vi "DG4DG1ZGeneral.vi"() -> ()   [LabVIEW 2020]
panel:
  out "output control error":errorcluster
  out "configure error out":errorcluster
  in  "Output 2":bool
  in  "Output 1":bool
  in  "Waveform Function":u16(ring)=1 items=["Sine", "Square", "Ramp", "Pulse", "Noise", "DC", "User"]
  in  "Channel Selection":u16(ring) items=["Channel 1", "Channel 2"]
  in  "Frequency (1000 Hz)":dbl=1000.0
  in  "Unit (0: Vpp)":u16(ring) items=["Vpp", "Vrms", "dB"]
  in  "DC Offset (0.00 V)":dbl
  in  "Amplitude (1)":dbl=1.0
  in  "?":bool
  in  "?":bool
  in  "VISA resource name":refnum<visa-resource-name>
  # "Rigol Technologies DG4/DG1Z General"
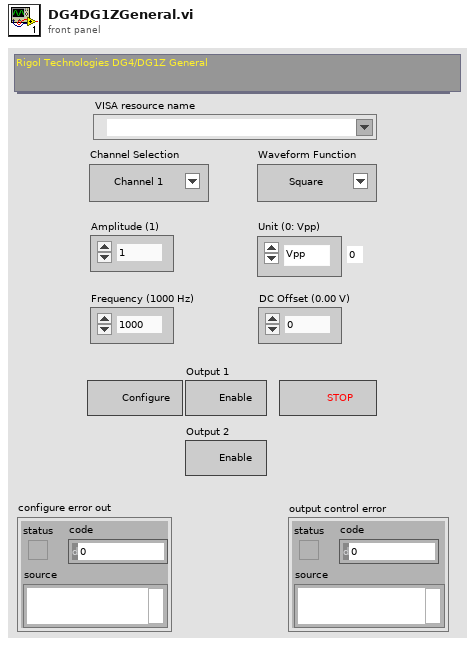
[diagram p1: front panel]
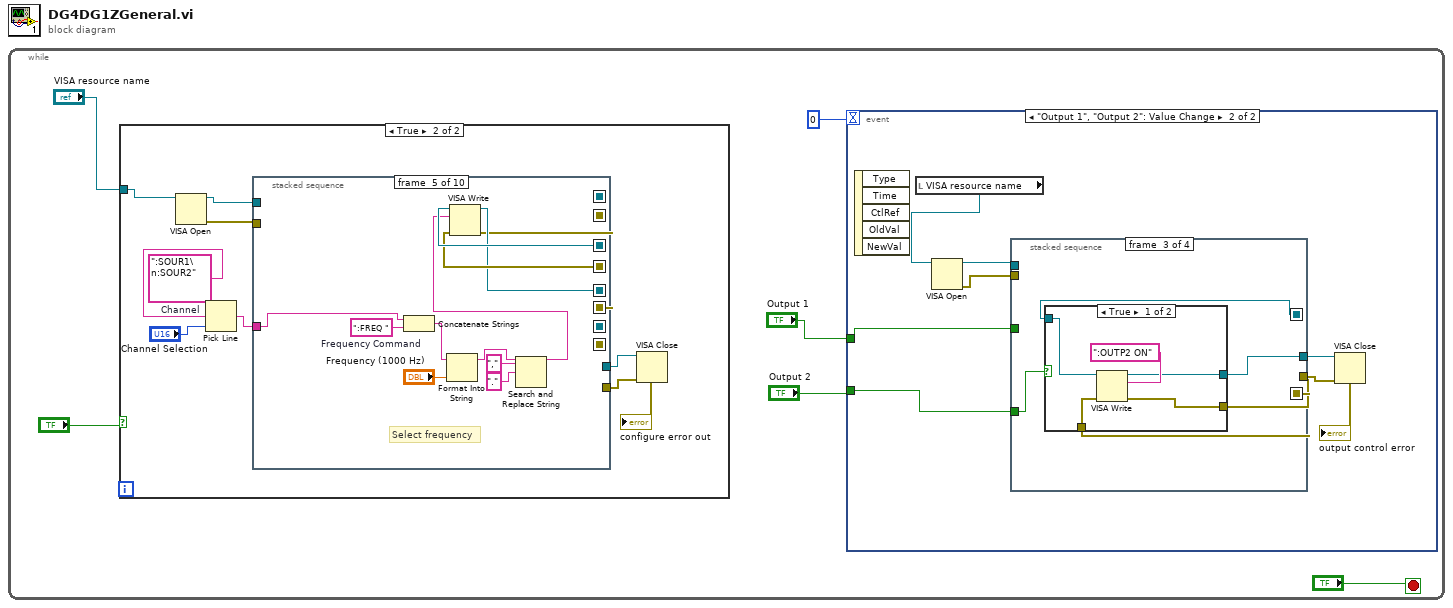
[diagram p0: block diagram]
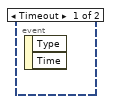
[diagram p2: hidden frame]
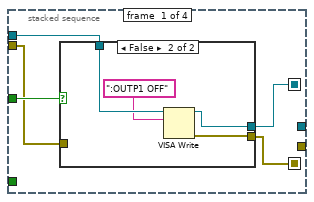
[diagram p3: hidden frame]
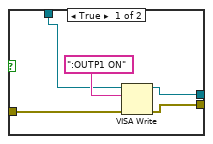
[diagram p4: hidden frame]
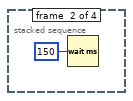
[diagram p5: hidden frame]
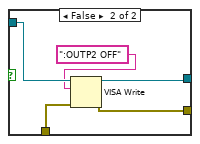
[diagram p6: hidden frame]
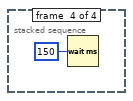
[diagram p7: hidden frame]
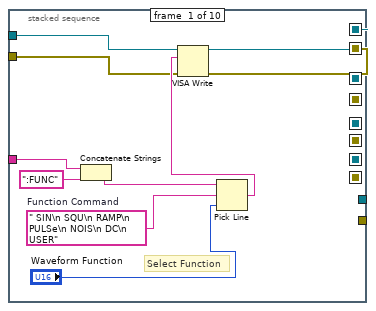
[diagram p9: hidden frame]
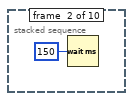
[diagram p10: hidden frame]
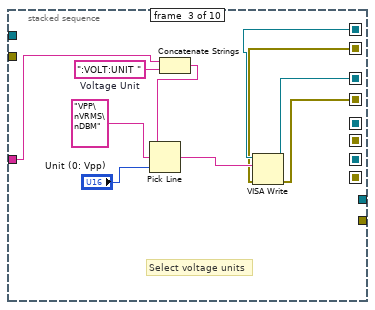
[diagram p11: hidden frame]
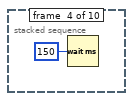
[diagram p12: hidden frame]
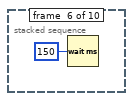
[diagram p13: hidden frame]
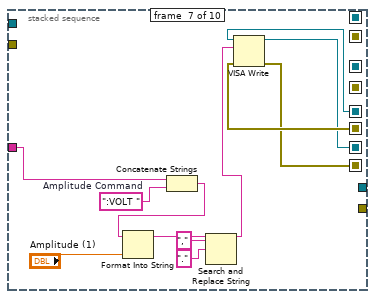
[diagram p14: hidden frame]
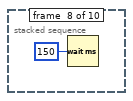
[diagram p15: hidden frame]
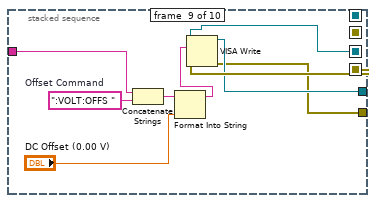
[diagram p16: hidden frame]
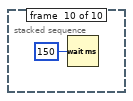
[diagram p17: hidden frame]
diagram:
  n1 = while {
    stop <- "?" stop-if-true
    n2 = case shown="True" "?" {
      tunnel: "VISA resource name" -> [_ w53]
      frame False {
      }
      frame True {
        w46 = ":SOUR1\n:SOUR2"  # Channel
        n3 = VISA Open(VISA resource name=w53) -> (VISA resource name=w52:refnum<visa-resource-name>, error out=w54:errorcluster)  [unwired: 4 in]
        n4 = Pick Line(multi-line string=w46, line index="Channel Selection") -> (output string=w48:string)  [unwired: 1 in]
        n5 = stacked-sequence {
          seq-local: [w58 _ _ _ _ _ _ _ _ _] -> [_ _ w70 _ _ _ _ _ _ _]
          seq-local: [w59 _ _ _ _ _ _ _ _ _] -> [_ _ w69 _ _ _ _ _ _ _]
          seq-local: [_ _ w68 _ _ _ _ _ _ _] -> [_ _ _ _ w85 _ _ _ _ _]
          seq-local: [_ _ w67 _ _ _ _ _ _ _] -> [_ _ _ _ w84 _ _ _ _ _]
          seq-local: [_ _ _ _ w83 _ _ _ _ _] -> [_ _ _ _ _ _ w98 _ _ _]
          seq-local: [_ _ _ _ w82 _ _ _ _ _] -> [_ _ _ _ _ _ w97 _ _ _]
          seq-local: [_ _ _ _ _ _ w96 _ _ _] -> [_ _ _ _ _ _ _ _ w107 _]
          seq-local: [_ _ _ _ _ _ w95 _ _ _] -> [_ _ _ _ _ _ _ _ w106 _]
          tunnel: w52 -> [w63 _ _ _ _ _ _ _ _ _]
          tunnel: w54 -> [w62 _ _ _ _ _ _ _ _ _]
          tunnel: [_ _ _ _ _ _ _ _ w105 _] -> w51
          tunnel: [_ _ _ _ _ _ _ _ w104 _] -> w50
          tunnel: w48 -> [w55 _ w66 _ w81 _ w94 _ w103 _]
          frame #0 {
            w57 = " SIN\n SQU\n RAMP\n PULSe\n NOIS\n DC\n USER"  # Function Command
            # "Select Function"
            n6 = Concatenate Strings(w55, ":FUNC" ("string (\"\")")) -> (w60:string)
            n7 = Pick Line(string ("")=w60, multi-line string=w57, line index="Waveform Function") -> (output string=w64:string)
            n8 = VISA Write(VISA resource name=w63, write buffer=w64, error in (no error)=w62) -> (VISA resource name out=w58:refnum<visa-resource-name>, error out=w59:errorcluster)  [unwired: 1 out]
          }
          frame #1 {
            n9 = Wait (ms)(milliseconds to wait=u32 150) -> ()  [unwired: 1 out]
          }
          frame #2 {
            w72 = ":VOLT:UNIT "  # Voltage Unit
            # "Select voltage units"
            n10 = Concatenate Strings(w66, w72) -> (w71:string)
            n11 = Pick Line(string ("")=w71, multi-line string="VPP\nVRMS\nDBM", line index="Unit (0: Vpp)") -> (output string=w74:string)
            n12 = VISA Write(VISA resource name=w70, write buffer=w74, error in (no error)=w69) -> (VISA resource name out=w68:refnum<visa-resource-name>, error out=w67:errorcluster)  [unwired: 1 out]
          }
          frame #3 {
            n13 = Wait (ms)(milliseconds to wait=u32 150) -> ()  [unwired: 1 out]
          }
          frame #4 {
            w87 = ":FREQ "  # Frequency Command
            # "Select frequency"
            n14 = Concatenate Strings(w81, w87) -> (w86:string)
            n15 = Format Into String(initial string=w86, "Frequency (1000 Hz)") -> (resulting string=w78:string)  [unwired: 2 in, 1 out]
            n16 = Search and Replace String(input string=w78, search string=",", replace string="." ("replace string (\"\")")) -> (result string=w77:string)  [unwired: 5 in, 3 out]
            n17 = VISA Write(VISA resource name=w85, write buffer=w77, error in (no error)=w84) -> (VISA resource name out=w83:refnum<visa-resource-name>, error out=w82:errorcluster)  [unwired: 1 out]
          }
          frame #5 {
            n18 = Wait (ms)(milliseconds to wait=u32 150) -> ()  [unwired: 1 out]
          }
          frame #6 {
            w100 = ":VOLT "  # Amplitude Command
            n19 = Concatenate Strings(w94, w100) -> (w99:string)
            n20 = Format Into String(initial string=w99, "Amplitude (1)") -> (resulting string=w93:string)  [unwired: 2 in, 1 out]
            n21 = Search and Replace String(input string=w93, search string=",", replace string="." ("replace string (\"\")")) -> (result string=w90:string)  [unwired: 5 in, 3 out]
            n22 = VISA Write(VISA resource name=w98, write buffer=w90, error in (no error)=w97) -> (VISA resource name out=w96:refnum<visa-resource-name>, error out=w95:errorcluster)  [unwired: 1 out]
          }
          frame #7 {
            n23 = Wait (ms)(milliseconds to wait=u32 150) -> ()  [unwired: 1 out]
          }
          frame #8 {
            w109 = ":VOLT:OFFS "  # Offset Command
            n24 = Concatenate Strings(w103, w109) -> (w108:string)
            n25 = Format Into String(initial string=w108, "DC Offset (0.00 V)") -> (resulting string=w111:string)  [unwired: 2 in, 1 out]
            n26 = VISA Write(VISA resource name=w107, write buffer=w111, error in (no error)=w106) -> (VISA resource name out=w105:refnum<visa-resource-name>, error out=w104:errorcluster)  [unwired: 1 out]
          }
          frame #9 {
            n27 = Wait (ms)(milliseconds to wait=u32 150) -> ()  [unwired: 1 out]
          }
        }
        n28 = VISA Close(VISA resource name=w51, error in (no error)=w50) -> (error out=→"configure error out":errorcluster)
      }
    }
    n29 = event shown="[1] \"Output 1\", \"Output 2\": Value Change" {
      selector: _ -> [_ _]
      dyn-events: _ -> [_ _]
      timeout: u32 0 ("Time") -> [_ _]
      tunnel: "Output 2" -> [_ w14]
      tunnel: "Output 1" -> [_ w13]
      event Timeout {
        n30 = event-data() -> ()  [unwired: 1 in, 2 out]
      }
      event "Output 1", "Output 2": Value Change {
        n31 = event-data() -> ()  [unwired: 1 in, 5 out]
        n32 = local read "VISA resource name"() -> (w12:refnum<visa-resource-name>)
        n33 = VISA Open(VISA resource name=w12) -> (VISA resource name=w11:refnum<visa-resource-name>, error out=w10:errorcluster)  [unwired: 4 in]
        n34 = stacked-sequence {
          seq-local: [w17 _ _ _] -> [_ _ w33 _]
          seq-local: [w15 _ _ _] -> [_ _ w31 _]
          tunnel: w11 -> [w19 _ _ _]
          tunnel: w14 -> [_ _ w34 _]
          tunnel: w13 -> [w18 _ _ _]
          tunnel: [_ _ w32 _] -> w9
          tunnel: w10 -> [w16 _ _ _]
          tunnel: [_ _ w30 _] -> w8
          frame #0 {
            n35 = case shown="False" w18 {
              tunnel: w19 -> [w23 w28]
              tunnel: [w22 w26] -> w17
              tunnel: w16 -> [w21 _]
              tunnel: [w20 w25] -> w15
              frame True {
                n36 = VISA Write(VISA resource name=w23, write buffer=":OUTP1 ON", error in (no error)=w21) -> (VISA resource name out=w20:refnum<visa-resource-name>, error out=w22:errorcluster)  [unwired: 1 out]
              }
              frame False {
                n37 = VISA Write(VISA resource name=w28, write buffer=":OUTP1 OFF") -> (VISA resource name out=w25:refnum<visa-resource-name>, error out=w26:errorcluster)  [unwired: 1 in, 1 out]
              }
            }
          }
          frame #1 {
            n38 = Wait (ms)(milliseconds to wait=u32 150) -> ()  [unwired: 1 out]
          }
          frame #2 {
            n39 = case shown="True" w34 {
              tunnel: w31 -> [w38 w44]
              tunnel: [w37 w42] -> w32
              tunnel: w33 -> [w36 w41]
              tunnel: [w35 w40] -> w30
              frame True {
                n40 = VISA Write(VISA resource name=w38, write buffer=":OUTP2 ON", error in (no error)=w36) -> (VISA resource name out=w35:refnum<visa-resource-name>, error out=w37:errorcluster)  [unwired: 1 out]
              }
              frame False {
                n41 = VISA Write(VISA resource name=w44, write buffer=":OUTP2 OFF", error in (no error)=w41) -> (VISA resource name out=w40:refnum<visa-resource-name>, error out=w42:errorcluster)  [unwired: 1 out]
              }
            }
          }
          frame #3 {
            n42 = Wait (ms)(milliseconds to wait=u32 150) -> ()  [unwired: 1 out]
          }
        }
        n43 = VISA Close(VISA resource name=w8, error in (no error)=w9) -> (error out=→"output control error":errorcluster)
      }
    }
  }
